vi "Get Name.vi"(8 "error in (no error)":errorcluster, 11 "DD Child B in":refnum<class "DD Child B.lvclass">) -> (0 "error out":errorcluster, 2 "name":string, 3 "DD Child B out":refnum<class "DD Child B.lvclass">)   [LabVIEW 2016, in "DD Child B.lvclass"]
uses:
  DD Child B.lvclass
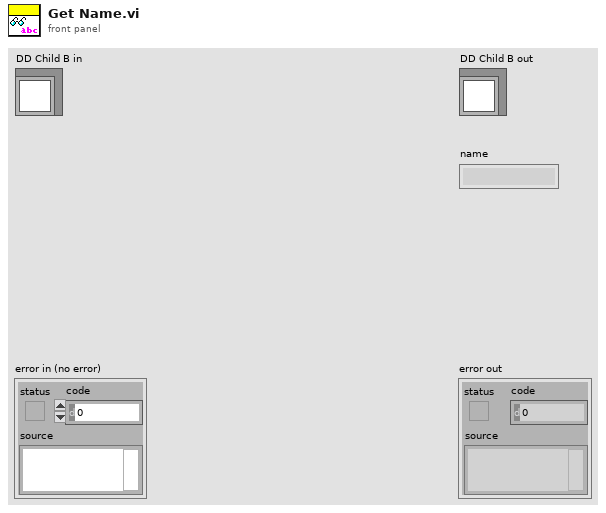
[diagram p1: front panel]
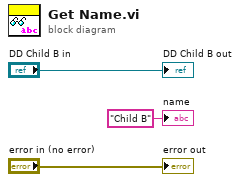
[diagram p0: block diagram]
diagram:
  "error out" <- "error in (no error)"
  "DD Child B out" <- "DD Child B in"
  "name" <- "Child B" ("name")
